vi "Df corr.vi"(5 "in":cdb[](array[numeric]), 9 "df":dbl) -> (8 "out":cdb[](array[numeric]))   [LabVIEW 2017]
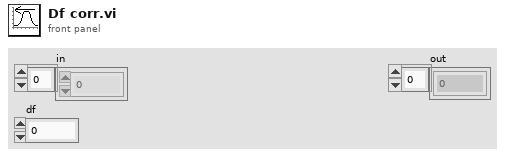
[diagram p1: front panel]
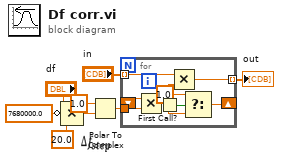
[diagram p0: block diagram]
diagram:
  n1 = Compound Arithmetic op=MULTIPLY("df", invert 7680000.0 ("value"), 20.0 ("y")) -> (w8:dbl)
  n2 = Polar To Complex(1:w8, 2:1.0 ("r")) -> (0:w7:cdb)
  n3 = for {
    tunnel: [w16] -> w4 mode=indexing
    tunnel: "in" -> [w15] mode=indexing
    shift-right: [w12] -> _
    shift-left: _ -> [w14]
    tunnel: w7 -> [w13]
    n4 = Multiply(x=w14, y=w13) -> (x*y=w10:cdb)
    n5 = First Call?() -> (First Call?: T/F=w11:bool)
    n6 = Multiply(x=w15, y=w10) -> (x*y=w16:cdb)
    n7 = Select(t=1.0, s=w11, f=w10) -> (s? t:f=w12:cdb)
  }
  "out" <- w4
